vi "Do.vi"(8 "error in (no error)":errorcluster, 10 "Actor in":refnum<class "Actor.lvclass">, 11 "Update Load Forecast Shortterm Msg":refnum<class "Update Load Forecast Shortterm Msg.lvclass">) -> (0 "error out":errorcluster, 2 "Actor out":refnum<class "Actor.lvclass">)   [LabVIEW 2016, in "Optimization Framework.lvlib" / "Update Load Forecast Shortterm Msg.lvclass"]
doc: "This VI delivers the message to the actor by calling the appropriate method(s) on the actor."
uses:
  Update Load Forecast Shortterm Msg.lvclass
  <vilib>/ActorFramework/Actor/Actor.lvclass
  Optimization/Optimization.lvclass
  C:/Program Files (x86)/National Instruments/LabVIEW 2016/vi.lib/ActorFramework/Actor/Actor.lvclass
  Update Load Forecast Shortterm Msg.lvclass/Update Load Forecast Shortterm Msg.ctl
  Optimization/Optimization.lvclass/Optimization.ctl
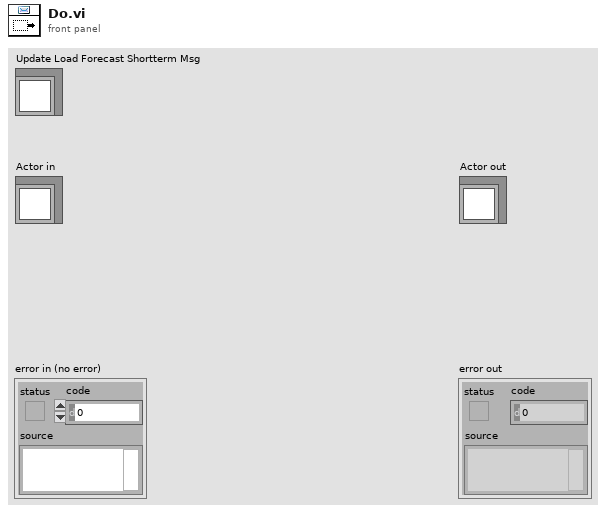
[diagram p1: front panel]
types:
  T1 = typedef "Optimization Framework.lvlib/Optimization.lvclass/Forecast Device Power.ctl" = cluster{"Device ID":u64, "t0":timestamp, "dt":dbl, "Power Array":dbl[], "Minimum Power Array":dbl[], "Maximum Power Array":dbl[], "PDF Array":T2[]}
  T2 = typedef "Optimization Framework.lvlib/Optimization.lvclass/PDF Cluster.ctl" = cluster{"P0":dbl, "dP":dbl, "Probability Array":dbl[]}
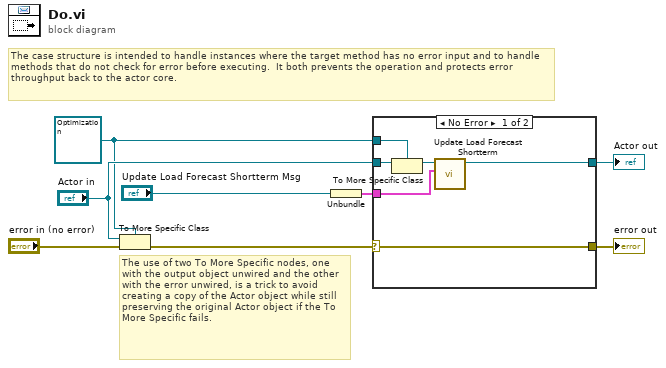
[diagram p0: block diagram]
diagram:
  w2 = refnum<class "Optimization.lvclass"> refnum ("Actor in")
  # "The use of two To More Specific nodes, one with the output object unwired and the other with the error unwired, is a trick to avoid creating a copy of the Actor object while still preserving the original Actor object if the To More Specific fails."
  # "The case structure is intended to handle instances where the target method has no error input and to handle methods that do not check for error before executing.  It both prevents the operation and protects error throughput back to the actor core."
  n1 = To More Specific Class(target class=w2, reference="Actor in", error in="error in (no error)") -> (error out=w6:errorcluster)  [unwired: 1 out]
  n2 = Unbundle("Update Load Forecast Shortterm Msg") -> (w1:T1)
  n3 = case shown="No Error" w6 {
    selector: w6 -> [w13 w16]
    tunnel: [w13 w16] -> w5
    tunnel: [w14 w15] -> w4
    tunnel: "Actor in" -> [w12 w15]
    tunnel: w2 -> [w11 _]
    tunnel: w1 -> [w9 _]
    frame No Error {
      n4 = To More Specific Class(target class=w11, reference=w12) -> (specific class reference=w10:refnum<class "Optimization.lvclass">)  [unwired: 1 in, 1 out]
      n5 = call "Update Load Forecast Shortterm.vi"("Load Power Forecast"=w9, "Optimization in"=w10) -> ("Optimization out"=w14:refnum<class "Optimization.lvclass">)  [unwired: 9 in]
    }
    frame Error {
      # "If type check fails, pass the original object out again."
    }
  }
  "error out" <- w5
  "Actor out" <- w4
